vi "Generate Workspace.vi"(8 "error in (no error)":errorcluster, 9 "XYZ Resolution":dbl[](array[numeric])=[0.01, 0.01, 0.01], 10 "Workspace Scope":T1={"X range"={"min"=-0.6, "max"=0.6}, "Y range"={"min"=-0.6, "max"=0.6}, "Z range"={"min"=-0.9, "max"=-0.4}}, 11 "Delta Analyzor in":refnum<class "Delta Analyzor.lvclass">) -> (0 "error out":errorcluster, 1 "number test points":i32, 2 "workspace":dbl[][](array[numeric]), 3 "Delta Analyzor out":refnum<class "Delta Analyzor.lvclass">)   [LabVIEW 2014, in "Delta Analyzor.lvclass"]
uses:
  Delta Analyzor.lvclass
  Workspace Scope.ctl
  Delta Analyzor.lvclass/Delta Analyzor.ctl
  Delta Robot Kinematics/Delta Robot Kinematics.lvclass
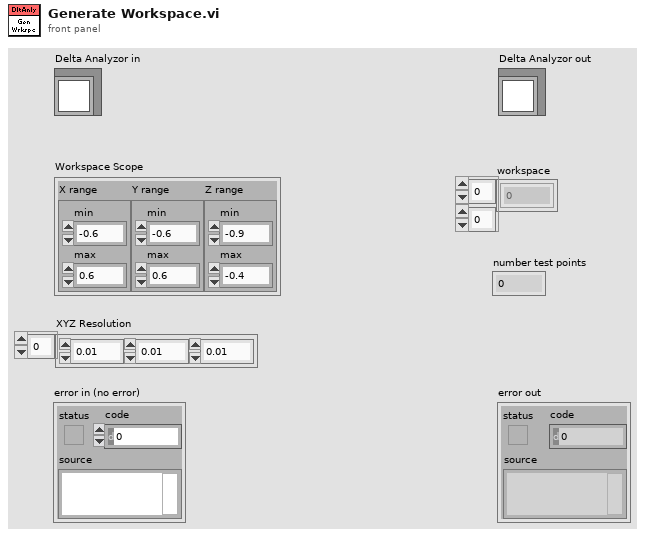
[diagram p1: front panel]
types:
  T1 = typedef "Delta Analyzor.lvclass/Workspace Scope.ctl" = cluster{"X range":cluster{"min":dbl, "max":dbl}, "Y range":cluster{"min":dbl, "max":dbl}, "Z range":cluster{"min":dbl, "max":dbl}}
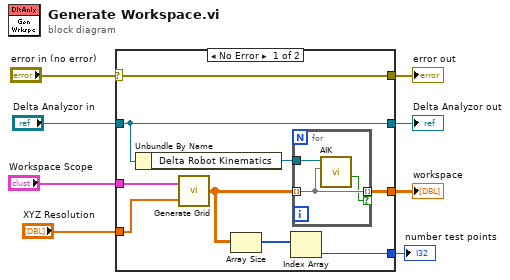
[diagram p0: block diagram]
diagram:
  n1 = case shown="No Error" "error in (no error)" {
    selector: "error in (no error)" -> [w17 w22]
    tunnel: [w17 w22] -> w7
    tunnel: [w16 w21] -> w5
    tunnel: "Delta Analyzor in" -> [w16 w21]
    tunnel: "Workspace Scope" -> [w15 _]
    tunnel: "XYZ Resolution" -> [w14 _]
    tunnel: [w12 _] -> w2
    tunnel: [w9 _] -> w1
    frame No Error {
      n2 = Unbundle By Name(w16) -> ("Delta Robot Kinematics"=w13:refnum<class "Delta Robot Kinematics.lvclass">)
      n3 = call "Generate Grid.vi"("XYZ Resolution"=w14, "Workspace Scope"=w15) -> ("grid points"=w11:dbl[][])
      n4 = Array Size(array=w11) -> (size(s)=w10:i32[])
      n5 = Index Array(array=w10) -> (element=w9:i32)  [unwired: 1 in]
      n6 = for {
        tunnel: w13 -> [w20]
        tunnel: w11 -> [w19] mode=indexing
        tunnel: [w19] -> w12 mode=indexing if=w18
        n7 = call-dynamic "AIK.vi"("p"=w19, "Delta Robot Kinematics in"=w20) -> ("exist"=w18:bool)  [unwired: 6 in, 3 out]
      }
    }
    frame Error {
    }
  }
  "error out" <- w7
  "Delta Analyzor out" <- w5
  "workspace" <- w2
  "number test points" <- w1
